vi "checkFinishStopOffensivePlay.vi"(8 "error in (no error)":errorcluster, 10 "Game":refnum<class "Game.lvclass">, 11 "StopOffensivePlay in":refnum<class "StopOffensivePlay.lvclass">) -> (0 "error out":errorcluster, 2 "Boolean":bool, 3 "StopOffensivePlay out":refnum<class "StopOffensivePlay.lvclass">)   [LabVIEW 2023, in "StopOffensivePlay.lvclass"]
uses:
  StopOffensivePlay.lvclass
  Game_class/Game.lvclass
  Referee_class/command_interpreted.ctl
  Game_class/Game.lvclass/Game.ctl
  Referee_class/Referee.lvclass/Referee.ctl
  Events_class/Events.lvclass/Events.ctl
  Game_class/Read Referee.vi
  Game_class/Read EventsRef.vi
  Events_class/Read ball_out.vi
  Referee_class/Read command_interpreted.vi
  Referee_class/Referee.lvclass
  Events_class/Events.lvclass
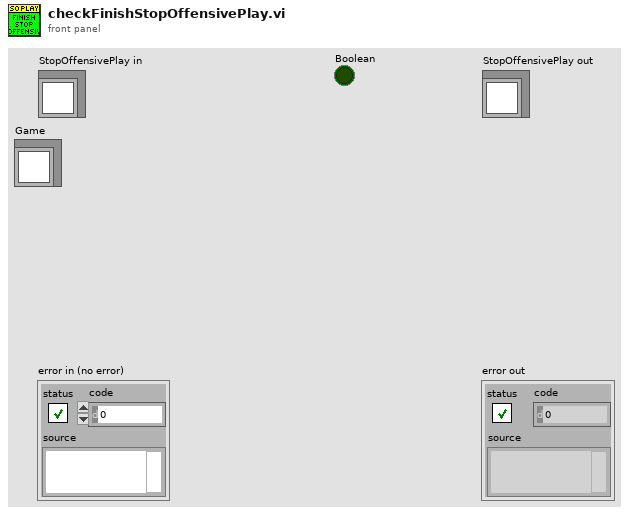
[diagram p1: front panel]
types:
  T1 = typedef "command_interpreted.ctl" = enum16{"Goal Ally", "Goal Enemy", "Ball Placement Enemy", "Ball Placement Ally", "Normal Half Time", "Extra Time  Break", "Extra Half Time", "None", "Post Game", "PKA Normal Start", "Prepare Kickoff Ally", "PKE Normal Start", "Prepare Kickoff Enemy", "Force Start", "Halt", "Timeout", "Prepare Penalty Ally", "Prepare Penalty Enemy", "PPA NormalStart", "PPE Normal Start", "Indirect Free Ally", "Direct Free Enemy", "Direct Free Ally", "Indirect Free Enemy", "Stop"}
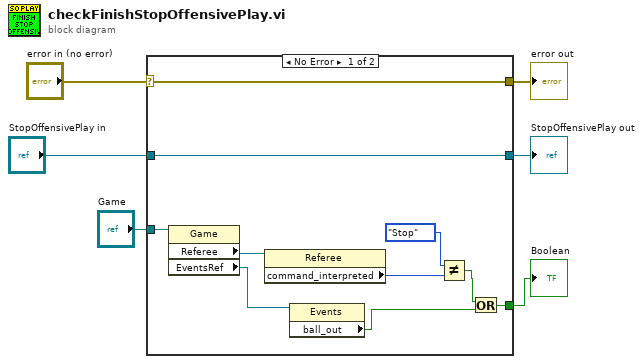
[diagram p0: block diagram]
diagram:
  n1 = case shown="No Error" "error in (no error)" {
    selector: "error in (no error)" -> [w15 w18]
    tunnel: [w15 w18] -> w5
    tunnel: [w16 w17] -> w3
    tunnel: "StopOffensivePlay in" -> [w16 w17]
    tunnel: "Game" -> [w13 _]
    tunnel: [w7 _] -> w1
    frame No Error {
      n2 = property class="Game"(reference=w13) -> ("Referee"=w14:refnum<class "Referee.lvclass">, "EventsRef"=w9:refnum<class "Events.lvclass">)  [unwired: 1 in, 2 out]
      n3 = property class="Referee"(reference=w14) -> ("command_interpreted"=w12:T1)  [unwired: 1 in, 2 out]
      n4 = property class="Events"(reference=w9) -> ("ball_out"=w8:bool)  [unwired: 1 in, 2 out]
      n5 = Not Equal?(x=command_interpreted."Stop" ("command_interpreted"), y=w12) -> (x != y?=w10:bool)
      n6 = Or(x=w10, y=w8) -> (x .or. y?=w7:bool)
    }
    frame Error {
    }
  }
  "error out" <- w5
  "StopOffensivePlay out" <- w3
  "Boolean" <- w1
